vi "Configure Null Function.vi"(6 "Enable Null Function (F: Disable)":bool, 7 "Auto Null Selection (T: Enable)":bool=TRUE, 8 "error in (no error)":errorcluster, 9 "Null Value (0)":dbl, 10 "Null Function Type (0: Current AC)":u16(ring) items=["Current AC", "Current DC", "Frequency", "Resistance 4-wire", "Period", "Resistance 2-wire", "Temperature", "Voltage AC", "Voltage DC", "Capacitance"], 11 "VISA resource name":refnum<visa-resource-name>) -> (0 "error out":errorcluster, 3 "VISA resource name out":refnum<visa-resource-name>)   [LabVIEW 2020, in "Agilent 3446X Series.lvlib"]
doc: "Configure null function settings for selected measurements.\n\n<b>Note(s):</b>\nThis vi is not supported for EDU34450A model."
uses:
  <instrlib>/Agilent 3446X Series/Agilent 3446X Series.lvlib
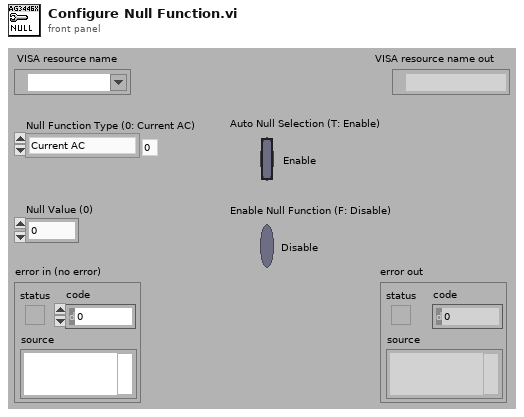
[diagram p1: front panel]
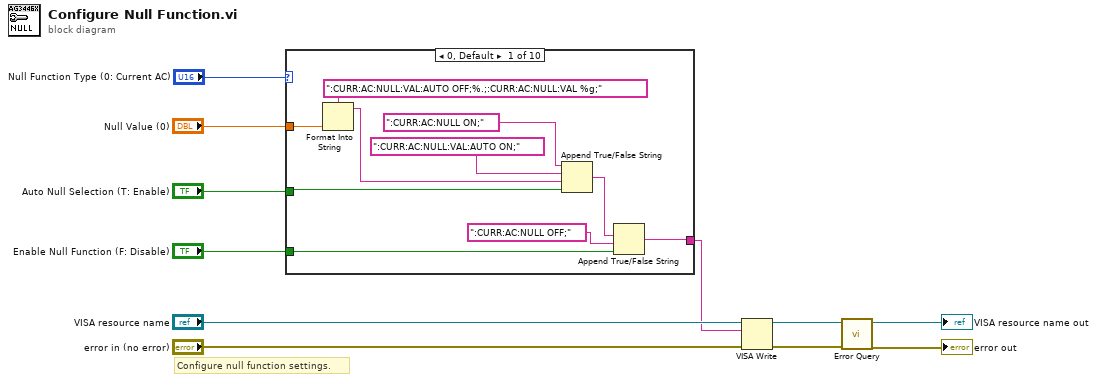
[diagram p0: block diagram]
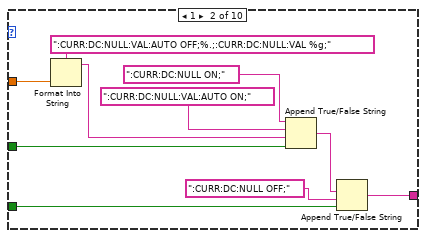
[diagram p2: hidden frame]
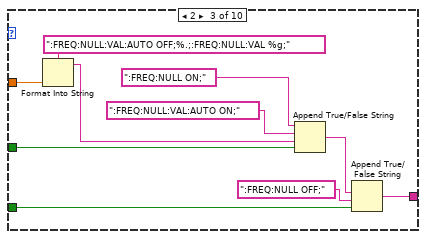
[diagram p3: hidden frame]
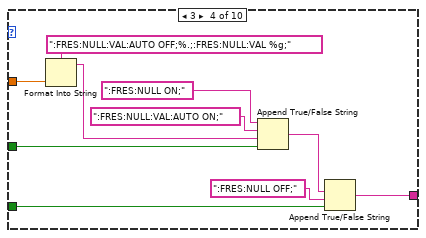
[diagram p4: hidden frame]
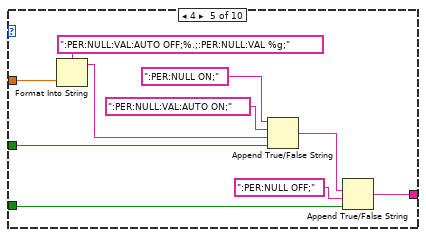
[diagram p5: hidden frame]
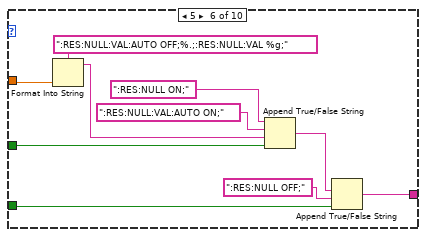
[diagram p6: hidden frame]
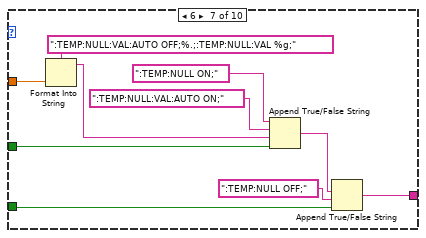
[diagram p7: hidden frame]
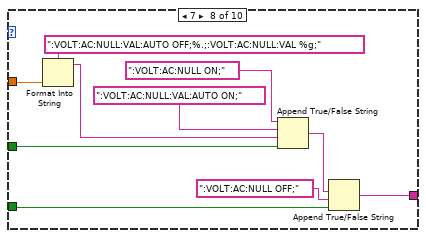
[diagram p8: hidden frame]
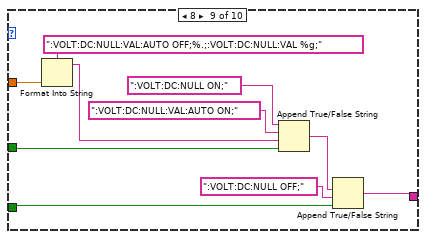
[diagram p9: hidden frame]
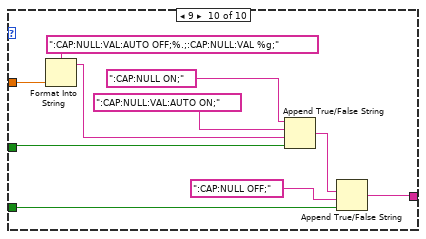
[diagram p10: hidden frame]
diagram:
  # "Configure null function settings."
  n1 = case shown="0, Default" "Null Function Type (0: Current AC)" {
    tunnel: [w15 w22 w35 w45 w55 w65 w75 w85 w95 w105] -> w1
    tunnel: "Null Value (0)" -> [w14 w25 w32 w42 w52 w62 w72 w82 w92 w104]
    tunnel: "Auto Null Selection (T: Enable)" -> [w13 w24 w33 w43 w53 w63 w73 w83 w93 w103]
    tunnel: "Enable Null Function (F: Disable)" -> [w12 w23 w34 w44 w54 w64 w74 w84 w94 w102]
    frame 0, Default {
      n2 = Format Into String(format string=":CURR:AC:NULL:VAL:AUTO OFF;%.;:CURR:AC:NULL:VAL %g;", w14) -> (resulting string=w19:string)  [unwired: 2 in, 1 out]
      n3 = Append True/False String(1:w13, 2:w19, 3:":CURR:AC:NULL:VAL:AUTO ON;", 4:":CURR:AC:NULL ON;") -> (0:w21:string)
      n4 = Append True/False String(1:w12, 2:":CURR:AC:NULL OFF;", 3:w21) -> (0:w15:string)  [unwired: 1 out]
    }
    frame 1 {
      n5 = Format Into String(format string=":CURR:DC:NULL:VAL:AUTO OFF;%.;:CURR:DC:NULL:VAL %g;", w25) -> (resulting string=w28:string)  [unwired: 2 in, 1 out]
      n6 = Append True/False String(1:w24, 2:w28, 3:":CURR:DC:NULL:VAL:AUTO ON;", 4:":CURR:DC:NULL ON;") -> (0:w26:string)
      n7 = Append True/False String(1:w23, 2:":CURR:DC:NULL OFF;", 3:w26) -> (0:w22:string)  [unwired: 1 out]
    }
    frame 2 {
      n8 = Format Into String(format string=":FREQ:NULL:VAL:AUTO OFF;%.;:FREQ:NULL:VAL %g;", w32) -> (resulting string=w38:string)  [unwired: 2 in, 1 out]
      n9 = Append True/False String(1:w33, 2:w38, 3:":FREQ:NULL:VAL:AUTO ON;", 4:":FREQ:NULL ON;") -> (0:w36:string)
      n10 = Append True/False String(1:w34, 2:":FREQ:NULL OFF;", 3:w36) -> (0:w35:string)  [unwired: 1 out]
    }
    frame 3 {
      n11 = Format Into String(format string=":FRES:NULL:VAL:AUTO OFF;%.;:FRES:NULL:VAL %g;", w42) -> (resulting string=w48:string)  [unwired: 2 in, 1 out]
      n12 = Append True/False String(1:w43, 2:w48, 3:":FRES:NULL:VAL:AUTO ON;", 4:":FRES:NULL ON;") -> (0:w46:string)
      n13 = Append True/False String(1:w44, 2:":FRES:NULL OFF;", 3:w46) -> (0:w45:string)  [unwired: 1 out]
    }
    frame 4 {
      n14 = Format Into String(format string=":PER:NULL:VAL:AUTO OFF;%.;:PER:NULL:VAL %g;", w52) -> (resulting string=w58:string)  [unwired: 2 in, 1 out]
      n15 = Append True/False String(1:w53, 2:w58, 3:":PER:NULL:VAL:AUTO ON;", 4:":PER:NULL ON;") -> (0:w56:string)
      n16 = Append True/False String(1:w54, 2:":PER:NULL OFF;", 3:w56) -> (0:w55:string)  [unwired: 1 out]
    }
    frame 5 {
      n17 = Format Into String(format string=":RES:NULL:VAL:AUTO OFF;%.;:RES:NULL:VAL %g;", w62) -> (resulting string=w68:string)  [unwired: 2 in, 1 out]
      n18 = Append True/False String(1:w63, 2:w68, 3:":RES:NULL:VAL:AUTO ON;", 4:":RES:NULL ON;") -> (0:w66:string)
      n19 = Append True/False String(1:w64, 2:":RES:NULL OFF;", 3:w66) -> (0:w65:string)  [unwired: 1 out]
    }
    frame 6 {
      n20 = Format Into String(format string=":TEMP:NULL:VAL:AUTO OFF;%.;:TEMP:NULL:VAL %g;", w72) -> (resulting string=w78:string)  [unwired: 2 in, 1 out]
      n21 = Append True/False String(1:w73, 2:w78, 3:":TEMP:NULL:VAL:AUTO ON;", 4:":TEMP:NULL ON;") -> (0:w76:string)
      n22 = Append True/False String(1:w74, 2:":TEMP:NULL OFF;", 3:w76) -> (0:w75:string)  [unwired: 1 out]
    }
    frame 7 {
      n23 = Format Into String(format string=":VOLT:AC:NULL:VAL:AUTO OFF;%.;:VOLT:AC:NULL:VAL %g;", w82) -> (resulting string=w88:string)  [unwired: 2 in, 1 out]
      n24 = Append True/False String(1:w83, 2:w88, 3:":VOLT:AC:NULL:VAL:AUTO ON;", 4:":VOLT:AC:NULL ON;") -> (0:w86:string)
      n25 = Append True/False String(1:w84, 2:":VOLT:AC:NULL OFF;", 3:w86) -> (0:w85:string)  [unwired: 1 out]
    }
    frame 8 {
      n26 = Format Into String(format string=":VOLT:DC:NULL:VAL:AUTO OFF;%.;:VOLT:DC:NULL:VAL %g;", w92) -> (resulting string=w98:string)  [unwired: 2 in, 1 out]
      n27 = Append True/False String(1:w93, 2:w98, 3:":VOLT:DC:NULL:VAL:AUTO ON;", 4:":VOLT:DC:NULL ON;") -> (0:w96:string)
      n28 = Append True/False String(1:w94, 2:":VOLT:DC:NULL OFF;", 3:w96) -> (0:w95:string)  [unwired: 1 out]
    }
    frame 9 {
      n29 = Format Into String(format string=":CAP:NULL:VAL:AUTO OFF;%.;:CAP:NULL:VAL %g;", w104) -> (resulting string=w109:string)  [unwired: 2 in, 1 out]
      n30 = Append True/False String(1:w103, 2:w109, 3:":CAP:NULL:VAL:AUTO ON;", 4:":CAP:NULL ON;") -> (0:w111:string)
      n31 = Append True/False String(1:w102, 2:":CAP:NULL OFF;", 3:w111) -> (0:w105:string)  [unwired: 1 out]
    }
  }
  n32 = VISA Write(VISA resource name="VISA resource name", write buffer=w1, error in (no error)="error in (no error)") -> (VISA resource name out=w9:refnum<visa-resource-name>, error out=w8:errorcluster)  [unwired: 1 out]
  n33 = call <instrlib>:"Error Query.vi"("error in (no error)"=w8, "VISA resource name"=w9) -> ("error out"=→"error out":errorcluster, "VISA resource name out"=→"VISA resource name out":refnum<visa-resource-name>)  [unwired: 8 out]
